vi "xor.vi"() -> ()   [LabVIEW 2016]
panel:
  out "a 3":i16
  out "a 2":i16
  out "a":i16
  in  "x 2":dbl
  in  "x1":dbl
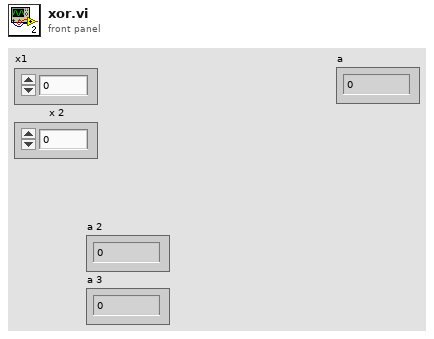
[diagram p1: front panel]
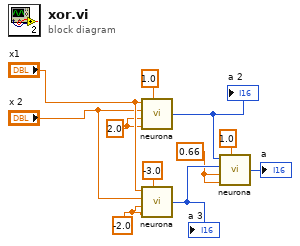
[diagram p0: block diagram]
diagram:
  w2 = 0.66 ("w 1")
  w7 = 2.0 ("w 1")
  w8 = -2.0 ("w 1")
  n1 = call "neurona.vi"("x1"="x1", "x 2"="x 2", "w 1"=w7, "w 2"=w7, "B"=1.0) -> ("a"=w4:i16)
  "a 2" <- w4
  n2 = call "neurona.vi"("x1"="x1", "x 2"="x 2", "w 1"=w8, "w 2"=w8, "B"=-3.0) -> ("a"=w3:i16)
  "a 3" <- w3
  n3 = call "neurona.vi"("x1"=w4, "x 2"=w3, "w 1"=w2, "w 2"=w2, "B"=1.0) -> ("a"=→"a":i16)
